vi "Write Control Function.vi"(8 "error in":errorcluster, 10 "Function":T1, 11 "MB_TCP session in":refnum<class "MB_Master_TCP.lvclass">) -> (0 "error out":errorcluster, 1 "Value":u16, 3 "MB session out":refnum<class "MB_Master_TCP.lvclass">)   [LabVIEW 2024, in "Bronkhorst Flexi-Flow ModbusTCP API.lvlib"]
uses:
  Bronkhorst Flexi-Flow ModbusTCP API.lvlib
  <vilib>/Plasmionique/MB Master/MB_Master_TCP/MB_Master_TCP.lvclass
  Control Function Values--enum.ctl
  PDU Address U16 Params--ring.ctl
  Write Unsigned Int Register.vi
  Read Unsigned Int Register.vi
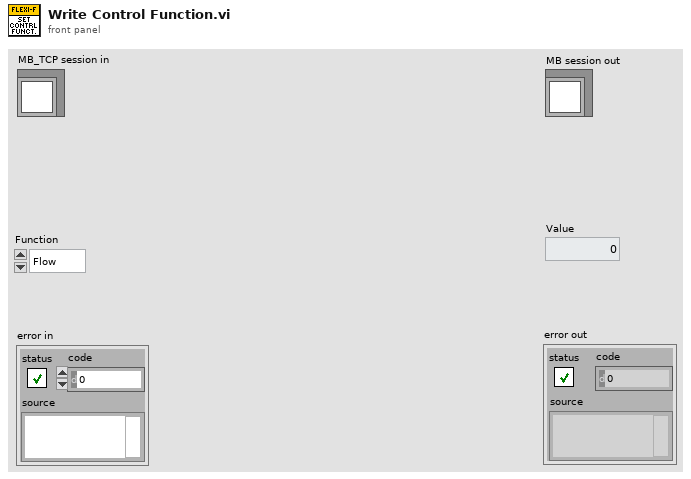
[diagram p1: front panel]
types:
  T1 = typedef "Bronkhorst Flexi-Flow ModbusTCP API.lvlib/Control Function Values--enum.ctl" = enum16{"Flow", "Upstream pressure", "Downstream pressure", "Flow with upstream pressure limit", "Flow with downstream pressure limit", "Upstream pressure with flow limit", "Downstream pressure with flow limit"}
  T2 = typedef "Bronkhorst Flexi-Flow ModbusTCP API.lvlib/PDU Address U16 Params--ring.ctl" = u16
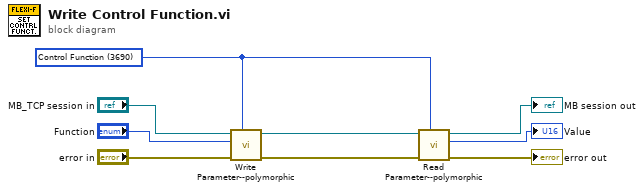
[diagram p0: block diagram]
diagram:
  w6 = T2 3690 items=["Setpoint"=33, "Setpoint slow"=34, "Alarm limit maximum"=3105, "Alarm limit minimum"=3106, "Alarm new setpoint"=3110, "Counter limit (UInt)"=3331, "Counter new setpoint"=3334, "Valve output"=61960, "Control Function"=3690, "TEMP"=0] ("PDU Address (U-Int16)")
  n1 = call-poly "Write Parameter--polymorphic.vi"("PDU Address (U-Int16)"=w6, "error in"="error in", "Value"="Function", "MB_TCP session in"="MB_TCP session in") -> ("error out"=w3:errorcluster, "MB session out"=w5:refnum<class "MB_Master_TCP.lvclass">)  [unwired: 6 in]
  n2 = call-poly "Read Parameter--polymorphic.vi"("PDU Address (U-Int16)"=w6, "error in"=w3, "MB_TCP session in"=w5) -> ("error out"=→"error out":errorcluster, "Value"=→"Value":u16, "MB session out"=→"MB session out":refnum<class "MB_Master_TCP.lvclass">)  [unwired: 6 in]
